vi "Add frames to send buffer.vi"(8 "error in (no error)":errorcluster, 10 "New Frame":T1 {"Data" format="%.0x"}, 11 "uCAN in":refnum<class "uCAN.lvclass">) -> (0 "error out":errorcluster, 3 "uCAN out":refnum<class "uCAN.lvclass">)   [LabVIEW 2021, in "uCanDriver.lvlib" / "uCAN.lvclass"]
uses:
  uCAN.lvclass
  typedefs/frame.ctl
  uCAN.lvclass/uCAN.ctl
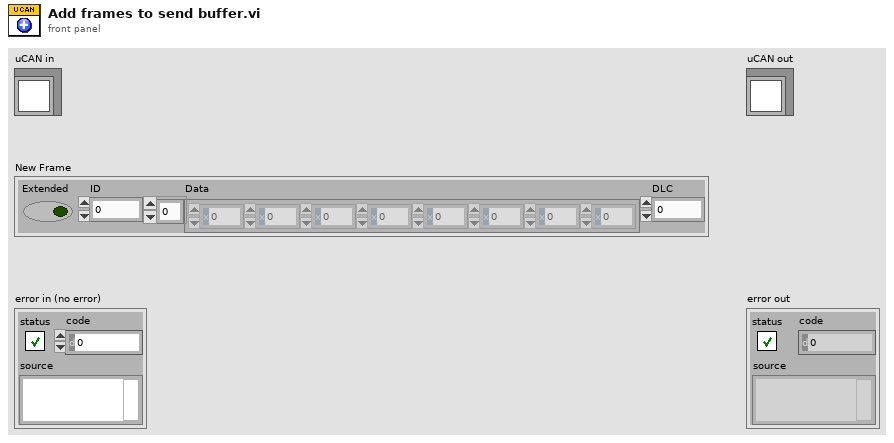
[diagram p1: front panel]
types:
  T1 = typedef "uCanDriver.lvlib/uCAN.lvclass/frame.ctl" = cluster{"Extended":bool, "ID":u32, "Data":u8[], "DLC":u8}
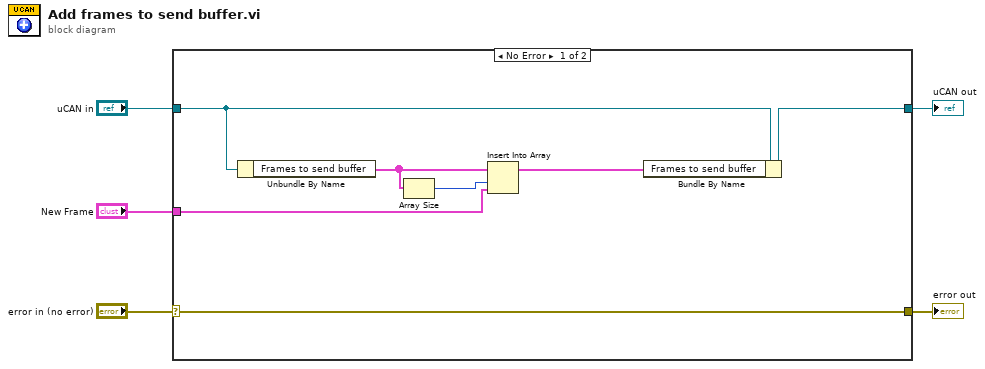
[diagram p0: block diagram]
diagram:
  n1 = case shown="No Error" "error in (no error)" {
    selector: "error in (no error)" -> [w12 w14]
    tunnel: [w12 w14] -> w4
    tunnel: [w11 w13] -> w2
    tunnel: "uCAN in" -> [w10 w13]
    tunnel: "New Frame" -> [w8 _]
    frame No Error {
      n2 = Unbundle By Name(w10) -> ("Frames to send buffer"=w7:T1[])
      n3 = Array Size(array=w7) -> (size(s)=w6:i32)
      n4 = Insert Into Array(array=w7, index=w6, new element=w8) -> (w9:T1[])
      n5 = Bundle By Name(cluster=w10, "Frames to send buffer"=w9) -> (w11:refnum<class "uCAN.lvclass">)
    }
    frame Error {
    }
  }
  "error out" <- w4
  "uCAN out" <- w2
